vi "frame2digits.vi"(1 "data from COM Port":string) -> (0 "Digits":u16[](array[numeric]))   [LabVIEW 2010]
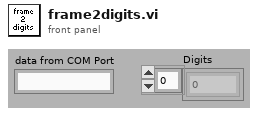
[diagram p1: front panel]
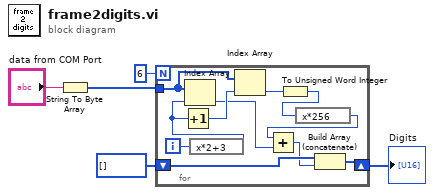
[diagram p0: block diagram]
diagram:
  n1 = String To Byte Array(string="data from COM Port") -> (unsigned byte array=w3:u8[])
  n2 = for {
    N: 6 -> [_]
    tunnel: w3 -> [w16]
    shift-right: [w12] -> w5
    shift-left: u16[] [] -> [w11]
    i -> [w15]
    n3 = expression code="x*2+3"(w15) -> (w13:i32)
    n4 = Increment(x=w13) -> (x+1=w14:i32)
    n5 = Index Array(array=w16, index=w13) -> (element=w6:u8)
    n6 = Index Array(array=w16, index=w14) -> (element=w9:u8)
    n7 = To Unsigned Word Integer(number=w9) -> (unsigned 16bit integer=w8:u16)
    n8 = expression code="x*256"(w8) -> (w7:u16)
    n9 = Add(x=w7, y=w6) -> (x+y=w10:u16)
    n10 = Build Array (concatenate)(w11, w10) -> (w12:u16[])
  }
  "Digits" <- w5
